vi "profibus to tag bus.vi"(9 "Data in":u8[](array[numeric]), 10 "slave configuration":T2, 11 "data table in":T1) -> (3 "data table out":T1)   [LabVIEW 2013, in "Profibus Module runtime.lvclass"]
uses:
  Profibus Module runtime.lvclass
  profibus slave configuration.ctl
  profibus mapping configuration.ctl
  <vilib>/NI/Tag Bus/tag/Data Type.ctl
  <vilib>/NI/Tag Bus/table/data table.ctl
  <vilib>/NI/Tag Bus/table/data polymorphs/write one/write Double.vi
  <vilib>/NI/Tag Bus/table/data polymorphs/write one/write Single.vi
  <vilib>/NI/Tag Bus/table/data polymorphs/write one/write Boolean.vi
  <vilib>/NI/Tag Bus/table/data table.lvlib
  <vilib>/NI/Tag Bus/tag/tag descriptor.lvclass
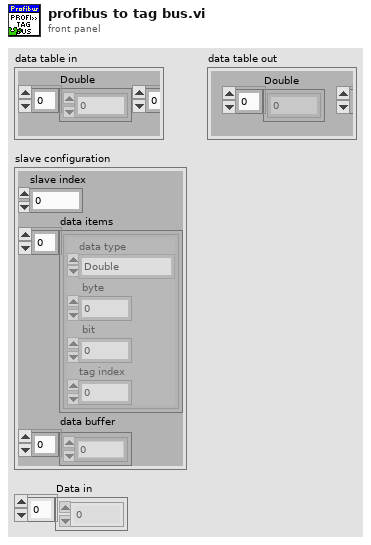
[diagram p1: front panel]
types:
  T1 = typedef "tag bus.lvlib/data table.lvlib/data table.ctl" = cluster{"Double":dbl[], "Single":sgl[], "I64":i64[], "I32":i32[], "I16":i16[], "I8":i8[], "U64":u64[], "U32":u32[], "U16":u16[], "U8":u8[], "Boolean":bool[], "String":string[], "Array of Double":cluster{"DBL Array":dbl[]}[], "Array of Single":cluster{"SGL Array":sgl[]}[], "Array of I64":cluster{"I64 Array":i64[]}[], "Array of I32":cluster{"I32 Array":i32[]}[], "Array of I16":cluster{"I16 Array":i16[]}[], "Array of I8":cluster{"I8 Array":i8[]}[], "Array of U64":cluster{"U64 Array":u64[]}[], "Array of U32":cluster{"U32 Array":u32[]}[], "Array of U16":cluster{"U16 Array":u16[]}[], "Array of U8":cluster{"U8 Array":u8[]}[], "Array of Boolean":cluster{"Boolean Array":bool[]}[], "Array of String":cluster{"String Array":string[]}[]}
  T2 = typedef "Profibus Module runtime.lvclass/profibus slave configuration.ctl" = cluster{"slave index":i8, "data items":T3[], "data buffer":u8[]}
  T3 = typedef "Profibus Module runtime.lvclass/profibus mapping configuration.ctl" = cluster{"data type":T4, " byte":i32, " bit":i32, "tag index":i32}
  T4 = typedef "tag bus.lvlib/tag descriptor.lvclass/Data Type.ctl" = enum16{"Double", "Single", "I64", "I32", "I16", "I8", "U64", "U32", "U16", "U8", "Boolean", "String", "Array of Double", "Array of Single", "Array of I64", "Array of I32", "Array of I16", "Array of I8", "Array of U64", "Array of U32", "Array of U16", "Array of U8", "Array of Boolean", "Array of String"}
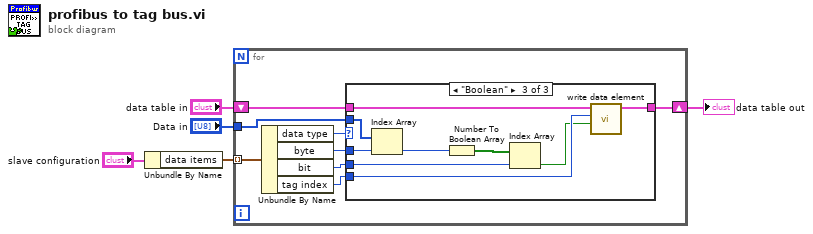
[diagram p0: block diagram]
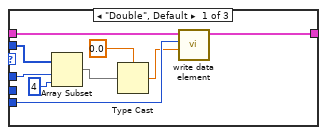
[diagram p2: hidden frame]
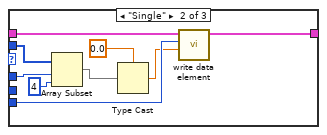
[diagram p3: hidden frame]
diagram:
  n1 = Unbundle By Name("slave configuration") -> ("data items"=w4:T3[])
  n2 = for {
    tunnel: w4 -> [w13] mode=indexing
    tunnel: "Data in" -> [w10]
    shift-right: [w7] -> w2
    shift-left: "data table in" -> [w6]
    n3 = Unbundle By Name(w13) -> ("data type"=w12:T4, "byte"=w11:i32, "bit"=w9:i32, "tag index"=w8:i32)
    n4 = case shown="\"Boolean\"" w12 {
      tunnel: w10 -> [w22 w31 w40]
      tunnel: w11 -> [w21 w30 w39]
      tunnel: w9 -> [_ _ w36]
      tunnel: w8 -> [w17 w26 w33]
      tunnel: [w15 w24 w35] -> w7
      tunnel: w6 -> [w14 w23 w34]
      frame "Double", Default {
        n5 = Array Subset(array=w22, index=w21, length=4) -> (w19:u8[])
        n6 = Type Cast(type=sgl 0.0, x=w19) -> (*(type *) &x=w16:sgl)
        n7 = call-poly <vilib>:"write data element.vi"("value"=w16, "index"=w17, "data table in"=w14) -> ("data table out"=w15:T1)  [unwired: 8 in]
      }
      frame "Single" {
        n8 = Array Subset(array=w31, index=w30, length=4) -> (w28:u8[])
        n9 = Type Cast(type=sgl 0.0, x=w28) -> (*(type *) &x=w25:sgl)
        n10 = call-poly <vilib>:"write data element.vi"("value"=w25, "index"=w26, "data table in"=w23) -> ("data table out"=w24:T1)  [unwired: 8 in]
      }
      frame "Boolean" {
        n11 = Index Array(array=w40, index=w39) -> (element=w38:u8)
        n12 = Number To Boolean Array(number=w38) -> (Boolean array=w37:bool[])
        n13 = Index Array(array=w37, index=w36) -> (element=w32:bool)
        n14 = call-poly <vilib>:"write data element.vi"("value"=w32, "index"=w33, "data table in"=w34) -> ("data table out"=w35:T1)  [unwired: 8 in]
      }
    }
  }
  "data table out" <- w2
